vi "Read Self Enqueuer.vi"(11 "Actor":refnum<class "Actor.lvclass">) -> (2 "Self Enqueuer":refnum<class "Message Enqueuer.lvclass">)   [LabVIEW 2020, in "Actor Framework.lvlib" / "Actor.lvclass"]
doc: "<p>(<strong>Filename</strong>: <span class=\"dnl\">Actor Framework.lvlib:Actor.lvclass:Read Self Enqueuer.vi</span>)</p>\n\n<p>Returns the reference needed for the actor to send messages to itself.</p>"
uses:
  Actor.lvclass
  Message Enqueuer/Message Enqueuer.lvclass
  Actor.lvclass/Actor.ctl
  Message Enqueuer/Message Enqueuer.lvclass/Message Enqueuer.ctl
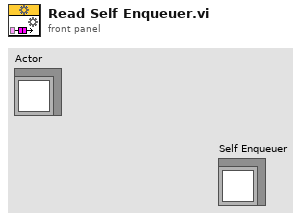
[diagram p1: front panel]
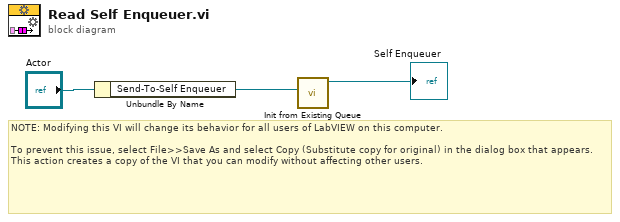
[diagram p0: block diagram]
diagram:
  # "NOTE: Modifying this VI will change its behavior for all users of LabVIEW on this computer.\n\nTo prevent this issue, select File>>Save As and select Copy (Substitute copy for original) in the dialog box that appears. This action creates a copy of the VI that you can modify without affecting other users."
  n1 = Unbundle By Name("Actor") -> ("Send-To-Self Enqueuer"=w1:refnum<class "Message Priority Queue.lvclass">)
  n2 = call "Init from Existing Queue.vi"("Priority Queue"=w1) -> ("Message Enqueuer"=→"Self Enqueuer":refnum<class "Message Enqueuer.lvclass">)  [unwired: 10 in]
